vi "set_triggerable_flag.vi"(8 "error in (no error)":errorcluster, 10 "triggerable?":bool, 11 "GenericSignalReader in":refnum<class "GenericSignalReader.lvclass">) -> (0 "error out":errorcluster, 3 "GenericSignalReader out":refnum<class "GenericSignalReader.lvclass">)   [LabVIEW 2010, in "GenericSignalReader.lvclass"]
uses:
  GenericSignalReader.lvclass
  GenericSignalReader.lvclass/GenericSignalReader.ctl
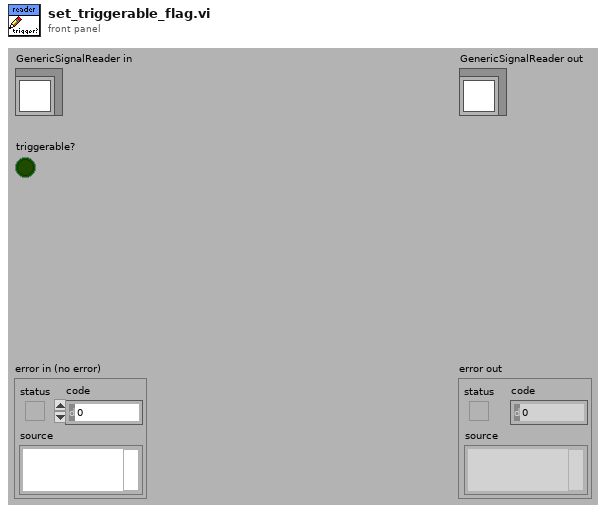
[diagram p1: front panel]
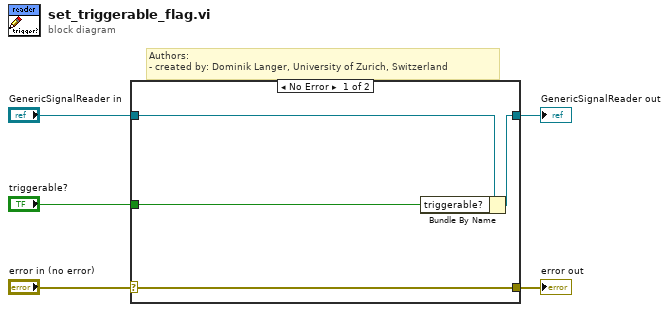
[diagram p0: block diagram]
diagram:
  # "Authors: \n- created by: Dominik Langer, University of Zurich, Switzerland"
  n1 = case shown="No Error" "error in (no error)" {
    selector: "error in (no error)" -> [w9 w10]
    tunnel: [w9 w10] -> w4
    tunnel: [w7 w11] -> w2
    tunnel: "GenericSignalReader in" -> [w8 w11]
    tunnel: "triggerable?" -> [w6 _]
    frame No Error {
      n2 = Bundle By Name(cluster=w8, "triggerable?"=w6) -> (w7:refnum<class "GenericSignalReader.lvclass">)
    }
    frame Error {
    }
  }
  "error out" <- w4
  "GenericSignalReader out" <- w2
